vi "Top Level VI Ref.vi"() -> (1 "Top Level VI reference":refnum<vi>)   [LabVIEW 2024, in "LVarex.lvlib"]
uses:
  LVarex.lvlib
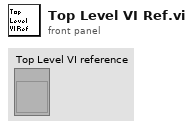
[diagram p1: front panel]
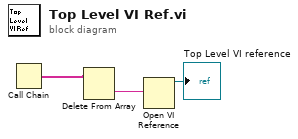
[diagram p0: block diagram]
diagram:
  n1 = Call Chain() -> (call chain=w3:string[])
  n2 = Delete From Array(array=w3) -> (deleted portion=w2:string)  [unwired: 2 in, 1 out]
  n3 = Open VI Reference(vi path=w2) -> (vi reference=→"Top Level VI reference":refnum<vi>)  [unwired: 5 in, 1 out]
